vi "get_partstudio_features.vi"(0 "Device In":T1, 11 "error in":errorcluster) -> (4 "Device Out":T1, 6 "Comm":T2, 15 "error out":errorcluster)   [LabVIEW 2019]
uses:
  <userlib>/IoT Devices/_subVIs/HTTPComm.ctl
  _SubVI/Cluster.ctl
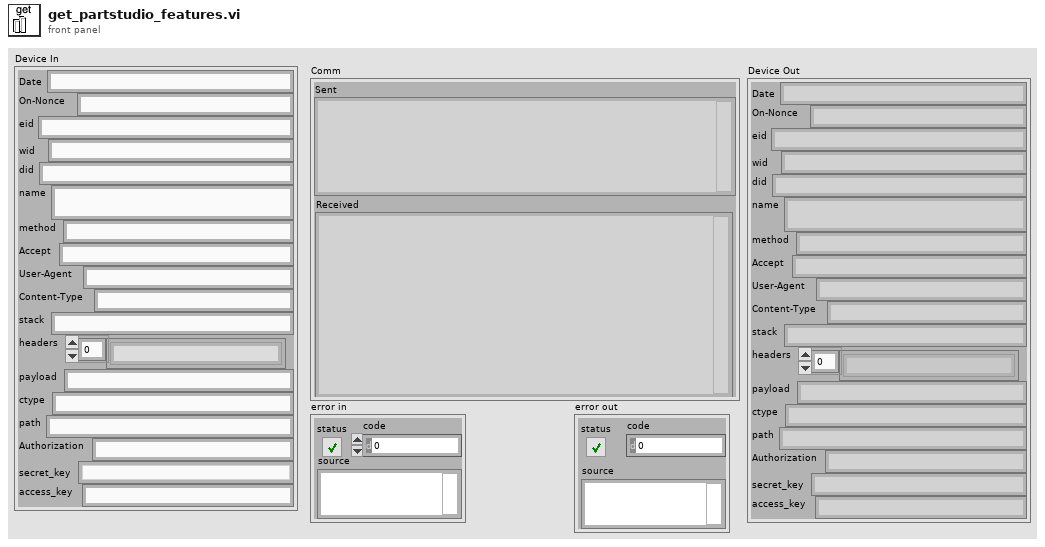
[diagram p1: front panel]
types:
  T1 = typedef "Cluster.ctl" = cluster{"Date":string, "On-Nonce":string, "eid":string, "wid":string, "did":string, "name":string, "method":string, "Accept":string, "User-Agent":string, "Content-Type":string, "stack":string, "headers":string[], "payload":string, "ctype":string, "path":string, "Authorization":string, "secret_key":string, "access_key":string}
  T2 = typedef "HTTPComm.ctl" = cluster{"url":string, "sent headers":string, "sent body":string, "headers":string, "body":string, "Sent":string, "Received":string}
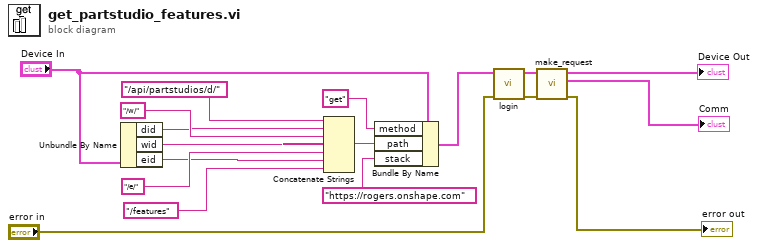
[diagram p0: block diagram]
diagram:
  n1 = Unbundle By Name("Device In") -> ("did"=w6:string, "wid"=w5:string, "eid"=w4:string)
  n2 = Concatenate Strings("/api/partstudios/d/" ("payload"), w6, "/w/" ("string"), w5, "/e/" ("string"), w4, "/features" ("string")) -> (w13:string)
  n3 = Bundle By Name(cluster="Device In", "method"="get" ("Method"), "path"=w13, "stack"="https://rogers.onshape.com" ("stacks")) -> (w1:T1)
  n4 = call "login.vi"("error in"="error in", "Device In"=w1) -> ("error out"=w8:errorcluster, "Device Out"=w11:T1)  [unwired: 8 in]
  n5 = call "make_request.vi"("Error in"=w8, "Device In"=w11) -> ("error out"=→"error out":errorcluster, "Comm"=→"Comm":T2, "Device Out"=→"Device Out":T1)  [unwired: 7 in]
